vi "SIM Min StepSize.vi"(1 "step size 2":dbl, 2 "step size 1":dbl) -> (0 "min step size":dbl)   [LabVIEW 2014]
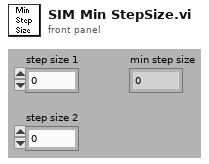
[diagram p1: front panel]
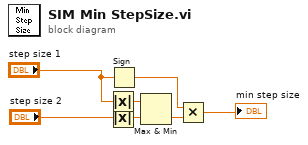
[diagram p0: block diagram]
diagram:
  n1 = Absolute Value(x="step size 1") -> (abs(x)=w4:dbl)
  n2 = Absolute Value(x="step size 2") -> (abs(x)=w3:dbl)
  n3 = Sign(1:"step size 1") -> (0:w5:dbl)
  n4 = Max & Min(x=w4, y=w3) -> (min(x,y)=w2:dbl)  [unwired: 1 out]
  n5 = Multiply(x=w5, y=w2) -> (x*y=→"min step size":dbl)
